vi "Move Contained Files to Folder.vi"(4 "Clear Empty Folder?(T)":bool=TRUE, 6 "exclued files":string[](array[string]), 8 "error in (no error)":errorcluster, 9 "overwrite (F)":bool=TRUE, 10 "Dest Foder Path":path, 11 "Folder Path":path) -> (0 "error out":errorcluster)   [LabVIEW 2017]
doc: "Moves the files directly inside Folder Path into Dest Foder Path, skipping the names listed in exclued files. Set overwrite (F) to replace existing files and Clear Empty Folder?(T) to delete source folders left empty."
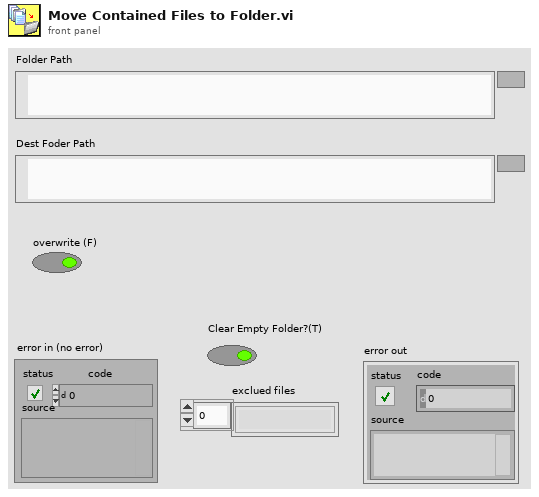
[diagram p1: front panel]
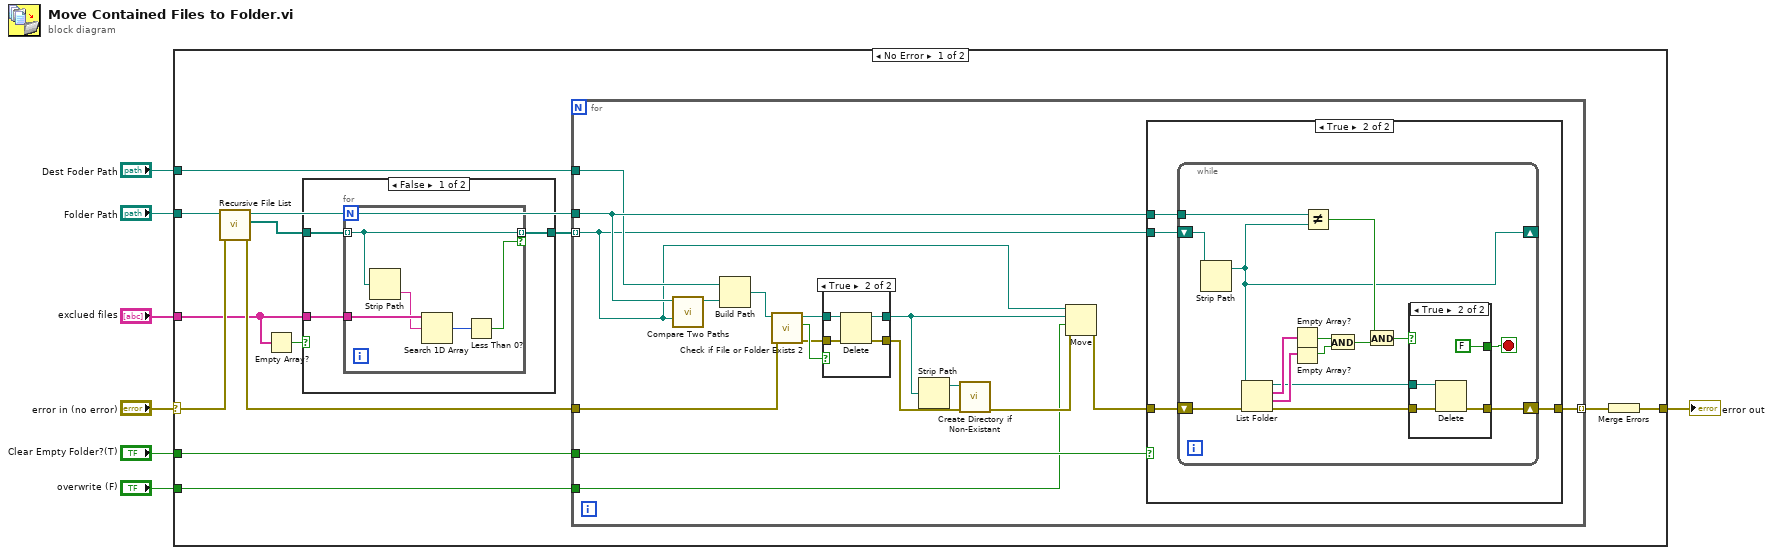
[diagram p0: block diagram]
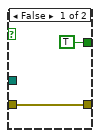
[diagram p4: hidden frame]
diagram:
  n1 = case shown="No Error" "error in (no error)" {
    selector: "error in (no error)" -> [w20 w79]
    tunnel: "Folder Path" -> [w18 _]
    tunnel: "Dest Foder Path" -> [w17 _]
    tunnel: [w14 w79] -> w4
    tunnel: "exclued files" -> [w13 _]
    tunnel: "Clear Empty Folder?(T)" -> [w9 _]
    tunnel: "overwrite (F)" -> [w8 _]
    frame No Error {
      n2 = call <vilib>:"Recursive File List.vi"("error in (no error)"=w20, "Folder Path"=w18) -> ("error out"=w19:errorcluster, "All Files in Dir"=w11:path[], "dup Folder Path"=w16:path)  [unwired: 5 in, 2 out]
      n3 = Empty Array?(array=w13) -> (empty?=w12:bool)
      n4 = case shown="False" w12 {
        tunnel: w13 -> [w23 _]
        tunnel: w11 -> [w22 w29]
        tunnel: [w21 w29] -> w10
        frame False {
          n5 = for {
            tunnel: w23 -> [w28]
            tunnel: w22 -> [w27] mode=indexing
            tunnel: [w27] -> w21 mode=indexing if=w24
            n6 = Strip Path(path=w27) -> (name=w26:string)  [unwired: 1 out]
            n7 = Search 1D Array(1D array=w28, element=w26) -> (index of element=w25:i32)  [unwired: 1 in]
            n8 = Less Than 0?(x=w25) -> (x < 0?=w24:bool)
          }
        }
        frame True {
        }
      }
      n9 = for {
        tunnel: w10 -> [w33] mode=indexing
        tunnel: w19 -> [w46]
        tunnel: w17 -> [w36]
        tunnel: w16 -> [w37]
        tunnel: [w34] -> w15 mode=indexing
        tunnel: w9 -> [w32]
        tunnel: w8 -> [w31]
        n10 = call <vilib>:"Compare Two Paths.vi"("Path 2"=w33, "Path 1"=w37) -> ("Relative Path from 1 to 2"=w30:path)  [unwired: 6 in, 3 out]
        n11 = Build Path(base path=w36, name or relative path=w30) -> (appended path=w45:path)
        n12 = call "Check if File or Folder Exists 2.vi"("error in (no error)"=w46, "path"=w45) -> ("error out"=w42:errorcluster, "file or folder exists?"=w43:bool, "dup path"=w44:path)  [unwired: 7 in]
        n13 = case shown="True" w43 {
          tunnel: w44 -> [w74 w78]
          tunnel: [w74 w77] -> w41
          tunnel: w42 -> [w73 w76]
          tunnel: [w73 w75] -> w39
          frame False {
          }
          frame True {
            n14 = Delete(path (use dialog)=w78, error in=w76) -> (deleted path=w77:path, error out=w75:errorcluster)  [unwired: 3 in, 1 out]
          }
        }
        n15 = Strip Path(path=w41) -> (stripped path=w40:path)  [unwired: 1 out]
        n16 = call "Create Directory if Non-Existant.vi"("error in (no error)"=w39, "Directory Path"=w40) -> ("error out"=w38:errorcluster)  [unwired: 7 in, 2 out]
        n17 = Move(source path=w33, error in=w38, 9:w31, 10:w41) -> (error out=w35:errorcluster)  [unwired: 1 in, 2 out]
        n18 = case shown="True" w32 {
          tunnel: w37 -> [_ w51]
          tunnel: w35 -> [w47 w50]
          tunnel: [w47 w49] -> w34
          tunnel: w33 -> [_ w48]
          frame False {
          }
          frame True {
            n19 = while {
              tunnel: w51 -> [w58]
              shift-right: [w54] -> w49
              shift-left: w50 -> [w55]
              shift-right: [w53] -> _
              shift-left: w48 -> [w59]
              stop <- w52 stop-if-true
              n20 = Strip Path(path=w59) -> (stripped path=w53:path)  [unwired: 1 out]
              n21 = List Folder(path=w53, error in=w55) -> (path out=w60:path, filenames=w66:string[], folder names=w65:string[], error out=w57:errorcluster)  [unwired: 2 in]
              n22 = Empty Array?(array=w66) -> (empty?=w64:bool)
              n23 = Empty Array?(array=w65) -> (empty?=w63:bool)
              n24 = Not Equal?(x=w58, y=w53) -> (x != y?=w61:bool)
              n25 = And(x=w64, y=w63) -> (x .and. y?=w62:bool)
              n26 = And(x=w61, y=w62) -> (x .and. y?=w56:bool)
              n27 = case shown="True" w56 {
                tunnel: w60 -> [_ w72]
                tunnel: w57 -> [w68 w71]
                tunnel: [w68 w70] -> w54
                tunnel: [TRUE FALSE] -> w52
                frame False {
                }
                frame True {
                  n28 = Delete(path (use dialog)=w72, error in=w71) -> (error out=w70:errorcluster)  [unwired: 3 in, 2 out]
                }
              }
            }
          }
        }
      }
      n29 = Merge Errors(w15) -> (w14:errorcluster)
    }
    frame Error {
    }
  }
  "error out" <- w4
